vi "New Image.vi"(8 "error in (no error)":errorcluster, 9 "Position":T1, 10 "File Path Control":path, 11 "Slide refnum in":refnum<k7>) -> (0 "error out":errorcluster, 2 "Picture refnum out":refnum<k7>, 3 "Slide refnum out":refnum<k7>)   [LabVIEW 2020, in "lvpptx.lvlib"]
uses:
  lvpptx.lvlib
  Position.ctl
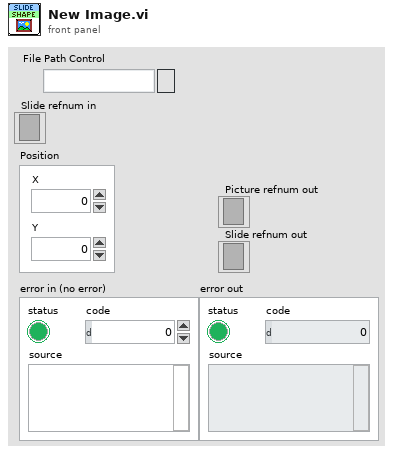
[diagram p1: front panel]
types:
  T1 = typedef "lvpptx.lvlib/Position.ctl" = cluster{"X":dbl, "Y":dbl}
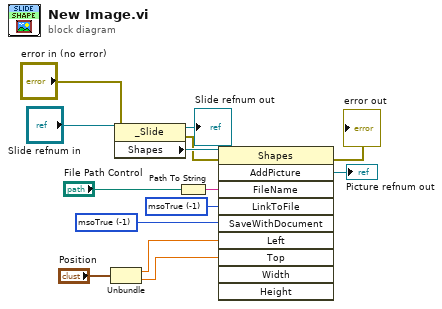
[diagram p0: block diagram]
diagram:
  w11 = -1 items=["msoTrue"=-1, "msoFalse"=0, "msoCTrue"=1, "msoTriStateToggle"=-3, "msoTriStateMixed"=-2] ("SaveWithDocument")
  w12 = -1 items=["msoTrue"=-1, "msoFalse"=0, "msoCTrue"=1, "msoTriStateToggle"=-3, "msoTriStateMixed"=-2] ("LinkToFile")
  n1 = Unbundle("Position") -> ("X"=w7:dbl, "Y"=w6:dbl)
  n2 = property class="_Slide"(reference="Slide refnum in", error in="error in (no error)") -> (reference out=→"Slide refnum out":refnum<k7>, error out=w13:errorcluster, "Shapes"=w14:refnum<k7>)
  n3 = Path To String(path="File Path Control") -> (string=w10:string)
  n4 = invoke class="Shapes" method="AddPicture"(reference=w14, error in=w13, "FileName"=w10, "LinkToFile"=w12, "SaveWithDocument"=w11, "Left"=w7, "Top"=w6) -> (error out=→"error out":errorcluster, "AddPicture"=→"Picture refnum out":refnum<k7>)  [unwired: 3 in, 8 out]
